vi "Start Arduino Comms.vi"(1 "Resource index":i32) -> (0 "Error":errorcluster)   [LabVIEW 2014]
uses:
  <vilib>/Instr/_visa.llb/VISA Open Access Mode.ctl
  Arduino_comms_Global.vi
  <vilib>/Instr/_visa.llb/VISA Configure Serial Port (Instr).vi
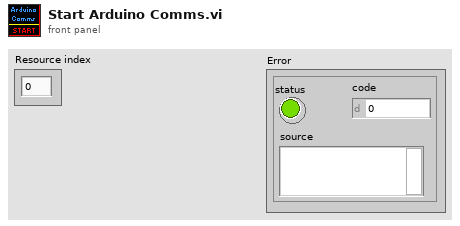
[diagram p1: front panel]
types:
  T1 = typedef "Arduino Config & resource typedef.ctl" = cluster{"VISA resource name":refnum<visa-resource-name>, "baud rate (bps)":u32, "timeout (ms)":u32, "data bits":u16, "parity":enum16{"None", "Odd", "Even", "Mark", "Space"}, "stop bits (10: 1 bit)":u16, "flow control":u16, "termination char (hex)":u8, "Enable Termination Char":bool, "byte count":u32, "Resource locked?":bool}
  T2 = typedef "VISA Open Access Mode.ctl" = u32
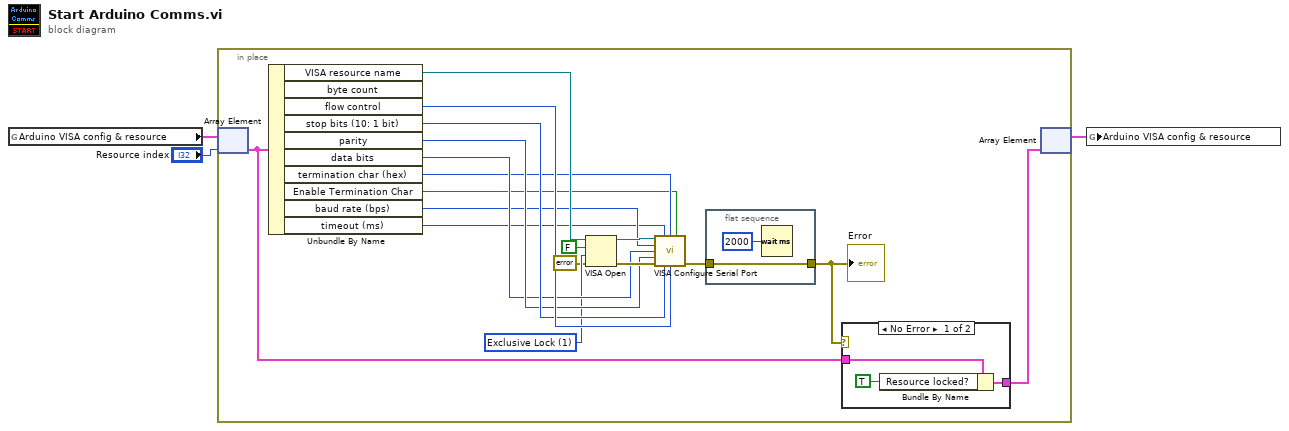
[diagram p0: block diagram]
diagram:
  n1 = global read "Arduino_comms_Global.vi" "Arduino VISA config & resource"() -> (w3:T1[])
  n2 = in-place {
    w10 = T2 1 items=["VISA Defaults"=0, "Exclusive Lock"=1, "Load Configured Settings"=4] ("Access Mode")
    n3 = in-place-array #1(w3, "Resource index") -> (w5:T1)
    n4 = Unbundle By Name(w5) -> ("VISA resource name"=w19:refnum<visa-resource-name>, "flow control"=w18:u16, "stop bits (10: 1 bit)"=w17:u16, "parity"=w16:enum16{"None", "Odd", "Even", "Mark", "Space"}, "data bits"=w15:u16, "termination char (hex)"=w12:u8, "Enable Termination Char"=w11:bool, "baud rate (bps)"=w14:u32, "timeout (ms)"=w13:u32)  [unwired: 1 out]
    n5 = VISA Open(duplicate session (F)=FALSE, access mode=w10, error in (no error)=errorcluster {"status"=FALSE, "code"=0, "source"=""}, VISA resource name=w19) -> (VISA resource name=w21:refnum<visa-resource-name>, error out=w20:errorcluster)  [unwired: 1 in]
    n6 = call-poly "VISA Configure Serial Port"("VISA resource name"=w21, "timeout (10sec)"=w13, "termination char\n(0xA = '\\n' = LF)"=w12, "Enable Termination\nChar (T)"=w11, "baud rate (9600)"=w14, "data bits (8)"=w15, "parity (0:none)"=w16, "error in (no error)"=w20, "stop bits (10: 1 bit)"=w17, "flow control (0:none)"=w18) -> ("error out"=w7:errorcluster)  [unwired: 4 in, 1 out]
    n7 = flat-sequence {
      tunnel: w7 -> [w22]
      tunnel: [w22] -> w6
      frame #0 {
        n8 = Wait (ms)(milliseconds to wait=u32 2000) -> ()  [unwired: 1 out]
      }
    }
    n9 = case shown="No Error" w6 {
      tunnel: [w24 w27] -> w4
      tunnel: w5 -> [w25 w27]
      frame No Error {
        n10 = Bundle By Name(cluster=w25, "Resource locked?"=TRUE ("Locked")) -> (w24:T1)
      }
      frame Error {
      }
    }
    n11 = in-place-array #1(w4) -> (w1:T1[])  [unwired: 1 out]
    "Error" <- w6
  }
  n12 = global write "Arduino_comms_Global.vi" "Arduino VISA config & resource"(w1) -> ()
